vi "GetAll_Tags_Units.vi"(8 "error in (no error)":errorcluster, 11 "FAMM in":refnum<class "FAMM.lvclass">) -> (0 "error out":errorcluster, 2 "Tags_Units":T1 {"EAQtagProps"."TagFunc" format="%08x"; "EAQtagProps"."RangeL" format="%.2f"; "EAQtagProps"."RangeH" format="%.2f"; "WAQtagProps"."TagFunc" format="%08x"; "WAQtagProps"."RangeL" format="%.2f"; "WAQtagProps"."RangeH" format="%.2f"; "PAQtagProps"."TagFunc" format="%08x"; "PAQtagProps"."RangeL" format="%.2f"; "PAQtagProps"."RangeH" format="%.2f"}, 3 "FAMM out":refnum<class "FAMM.lvclass">)   [LabVIEW 2020, in "FAMM.lvclass"]
doc: "Read Tags and Engineering units (and other TAG properties) from FAMM"
uses:
  FAMM.lvclass
  controls/Typedef_Gviewer_TagsUnits.ctl
  Common/controls/typedef_com_TagProp.ctl
  FAMM.lvclass/FAMM.ctl
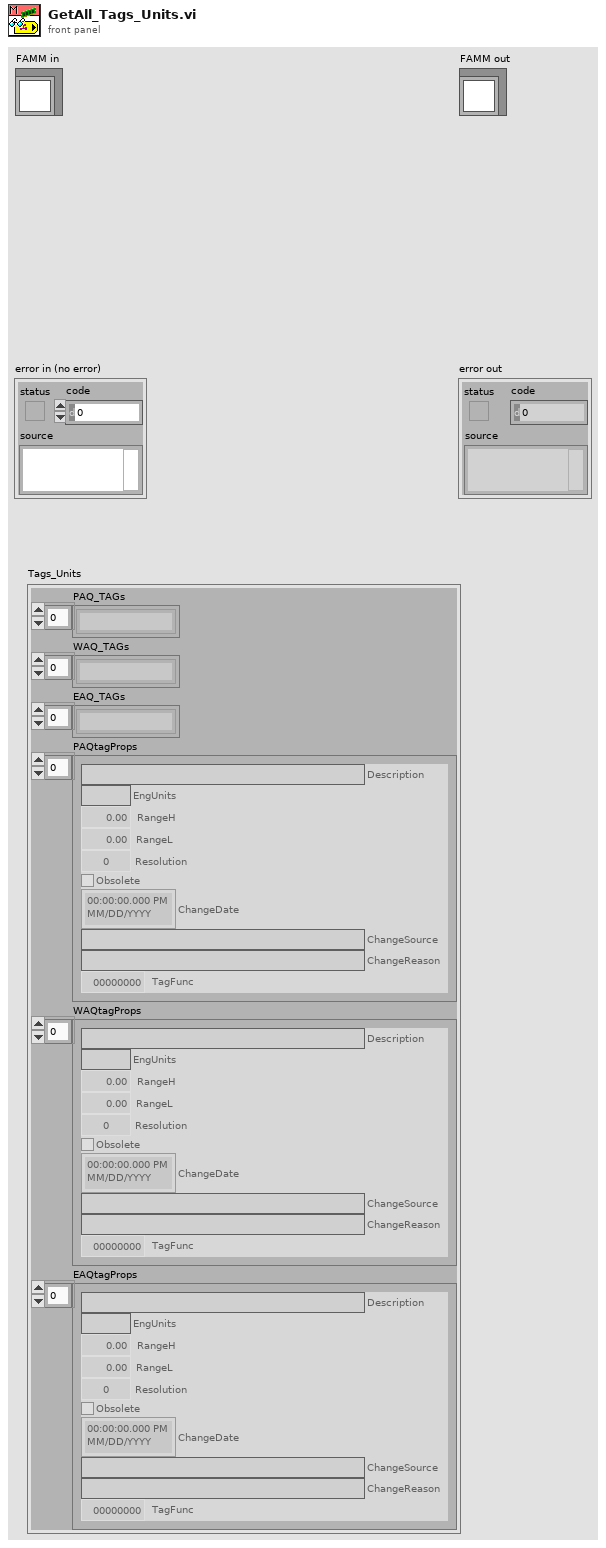
[diagram p1: front panel]
types:
  T1 = typedef "FAMM.lvclass/Typedef_Gviewer_TagsUnits.ctl" = cluster{"PAQ_TAGs":string[], "WAQ_TAGs":string[], "EAQ_TAGs":string[], "PAQtagProps":T2[], "WAQtagProps":T2[], "EAQtagProps":T2[]}
  T2 = typedef "typedef_com_TagProp.ctl" = cluster{"Description":string, "EngUnits":string, "RangeH":dbl, "RangeL":dbl, "Resolution":i32, "Obsolete":bool, "ChangeDate":timestamp, "ChangeSource":string, "ChangeReason":string, "TagFunc":u32}
  T3 = typedef "FAMM.lvclass/FAMM-attributes.ctl" = cluster{"FAMM_PAQ_Layers":i32, "FAMM_PAQ_resolution":dbl, "PAQ_TAGs":string[], "WAQ_TAGs":string[], "EAQ_TAGs":string[], "All_TAGs":string[], "PAQtagProps":T2[], "WAQtagProps":T2[], "EAQtagProps":T2[], "DBAL_class":refnum<data-value>, "PAQ_memory":refnum<data-value>[], "PAQupdates":timestamp[], "FAMM_Size":cluster{"other":i32, "1day":i32, "1week":i32}, "DatabaseFileExtention":string, "DatabaseSaveRate":dbl, "Database_path":path}
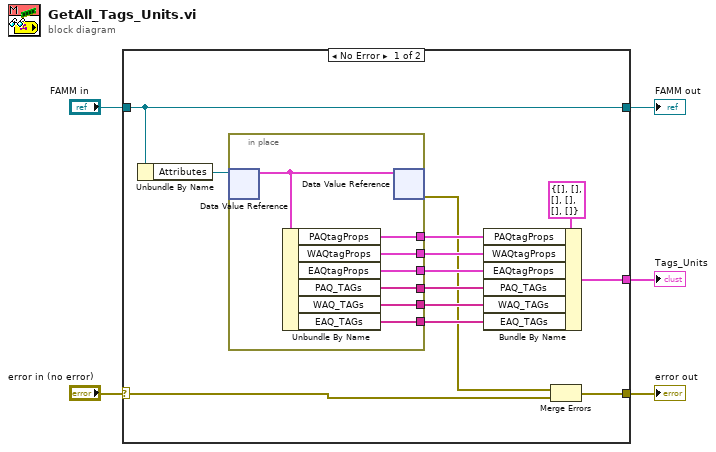
[diagram p0: block diagram]
diagram:
  n1 = case shown="No Error" "error in (no error)" {
    selector: "error in (no error)" -> [w7 w26]
    tunnel: [w6 w26] -> w4
    tunnel: [w18 w27] -> w2
    tunnel: "FAMM in" -> [w18 w27]
    tunnel: [w9 _] -> w1
    frame No Error {
      n2 = Unbundle By Name(w18) -> ("Attributes"=w17:refnum<data-value>)
      n3 = in-place {
        in-place-border: [w24] -> w15
        in-place-border: [w23] -> w14
        in-place-border: [w22] -> w13
        in-place-border: [w21] -> w12
        in-place-border: [w20] -> w11
        in-place-border: [w19] -> w10
        n4 = in-place-dvr #1(w17) -> (w25:T3)  [unwired: 1 out]
        n5 = Unbundle By Name(w25) -> ("PAQtagProps"=w24:T2[], "WAQtagProps"=w23:T2[], "EAQtagProps"=w22:T2[], "PAQ_TAGs"=w21:string[], "WAQ_TAGs"=w20:string[], "EAQ_TAGs"=w19:string[])
        n6 = in-place-dvr #1(w25) -> (w8:errorcluster)  [unwired: 1 out]
      }
      n7 = Bundle By Name(cluster=T1 {"PAQ_TAGs"=[], "WAQ_TAGs"=[], "EAQ_TAGs"=[], "PAQtagProps"=[], "WAQtagProps"=[], "EAQtagProps"=[]} ("Tags_Units"), "PAQtagProps"=w15, "WAQtagProps"=w14, "EAQtagProps"=w13, "PAQ_TAGs"=w12, "WAQ_TAGs"=w11, "EAQ_TAGs"=w10) -> (w9:T1)
      n8 = Merge Errors(w8, w7) -> (w6:errorcluster)
    }
    frame Error {
    }
  }
  "error out" <- w4
  "FAMM out" <- w2
  "Tags_Units" <- w1
